vi "Multi_spectra.vi"(7 "Equi Spaced":dbl[][](array[numeric]) format="%.2f") -> (3 "Spectra":dbl[][](array[numeric]) format="%.2f")   [LabVIEW 2010]
uses:
  Globals/Meas_global.vi
  Globals/LDA_meas_global_1.vi
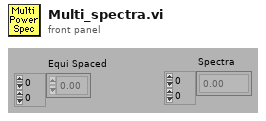
[diagram p1: front panel]
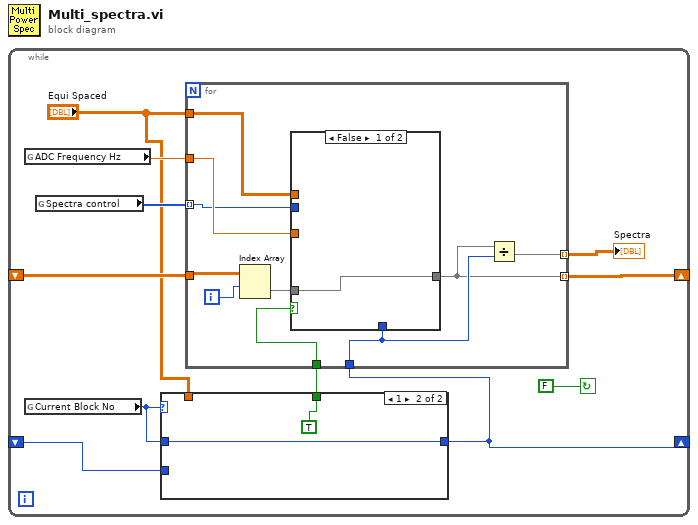
[diagram p0: block diagram]
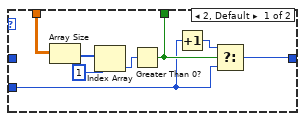
[diagram p2: hidden frame]
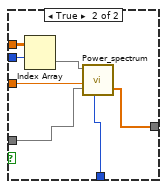
[diagram p3: hidden frame]
diagram:
  n1 = while {
    shift-left: _ -> [w8]
    shift-right: [w10] -> _
    shift-right: [w4] -> _
    shift-left: _ -> [w1]
    stop <- FALSE continue-if-true
    n2 = global read "LDA_meas_global_1.vi" "ADC Frequency Hz"() -> (w7:dbl)
    n3 = global read "Meas_global.vi" "Current Block No"() -> (w5:i32)
    n4 = global read "Meas_global.vi" "Spectra control"() -> (w9:i32[])
    n5 = case shown="1" w5 {
      tunnel: [w12 w21] -> w4
      tunnel: w5 -> [_ w21]
      tunnel: "Equi Spaced" -> [w19 _]
      tunnel: [w15 TRUE] -> w2
      tunnel: w1 -> [w13 _]
      frame 2, Default {
        n6 = Array Size(array=w19) -> (size(s)=w18:i32[])
        n7 = Index Array(array=w18, index=1) -> (element=w16:i32)
        n8 = Greater Than 0?(x=w16) -> (x > 0?=w15:bool)
        n9 = Increment(x=w13) -> (x+1=w14:i32)
        n10 = Select(t=w14, s=w15, f=w13) -> (s? t:f=w12:i32)
      }
      frame 1 {
      }
    }
    n11 = for {
      tunnel: w9 -> [w28] mode=indexing
      tunnel: "Equi Spaced" -> [w29]
      tunnel: w7 -> [w31]
      tunnel: [w23] -> w11 mode=indexing
      tunnel: w4 -> [w30]
      tunnel: [w22] -> w10 mode=indexing
      tunnel: w8 -> [w25]
      tunnel: w2 -> [w27]
      i -> [w26]
      n12 = Index Array(array=w25, index (row)=w26) -> (element=w24:dbl[])  [unwired: 1 in]
      n13 = case shown="False" w27 {
        tunnel: w31 -> [_ w39]
        tunnel: w30 -> [_ w38]
        tunnel: [w32 w37] -> w22
        tunnel: w29 -> [_ w36]
        tunnel: w28 -> [_ w35]
        tunnel: w24 -> [w32 w33]
        frame False {
        }
        frame True {
          n14 = Index Array(array=w36, index (row)=w35) -> (element=w34:dbl[])  [unwired: 1 in]
          n15 = call "Power_spectrum.vi"("U"=w34, "Sampling frequency"=w39, "Spectrum input array"=w33, "Block No"=w38) -> ("Spectrum output array"=w37:dbl[])  [unwired: 1 in, 1 out]
        }
      }
      n16 = Divide(x=w22, y=w30) -> (x/y=w23:dbl[])
    }
    "Spectra" <- w11
  }
